vi "HW Configuration Dialog.vi"(8 "error in (no error)":errorcluster, 11 "Settings in":T2={"Support"={"Save Configuration"={"Log File Base Path"=path "", "TDMS File Reference"=refnum, "Reset"=FALSE, "Wait"=0.0, "Start Time"=0.0, "Update Rate"=1, "Channel Names"=[], "System Preset"=variant}, "LOG Configuration"={"LOG REF"=refnum, "Writer Queue"=refnum, "Log Path"=path "", "LOG"=FALSE}, "ALARM Configuration"={"LOG REF"=refnum, "Writer Queue"=refnum, "Log Path"=path "", "UPS standby"=FALSE, "status code"=5001, "SP"=[], "Over Sens Status"=[]}, "User Details"=[], "Radome Type"="", "Timer Configuration"={"Wait"=0.0, "Next Step"="", "Writer Queue"=refnum, "Reset"=FALSE, "VISA resource"="", "Status"=[], "Valve Time"=[], "Timer queue"=refnum, "Current valve"=0, "Enable"=FALSE}}, "Process"={"Test Configuration"={"current Step"=0, "Wait"=0.0, "Next Step"="", "Writer Queue"=refnum, "Reset"=FALSE, "SEQ Time"=0, "General Reset"=FALSE, "Cycles"=0, "Status"=[], "Ready"=[], "Backward"=FALSE, "Current SP"=[], "System Preset"={"Test Configuration"={"Cycles"=0, "Z Up"=0.0, "SP List"=[], "Operator"="", "Point Delay"=0, "Z Up 2"=0.0, "Cleaning In"=0.0, "Cleaning Out"=0.0, "Cleaning Cycles"=0}, "Test_Start_date"=""}, "Test Type"=enum."Calibration", "Sample Count"=0, "Local Queues"={"Cycles queue"=refnum, "Step queue"=refnum, "RES Queue"=refnum, "Clean queue"=refnum, "PS Scan queue"=refnum}, "current Clean"=0, "PS Measure Plan"=[]}}, "Report Configuration"={"Test Setting"={"Test_Num"=0, "Test_ID"=0, "Proc_ID"=0, "Max Force"=0.0, "User"="", "SN"="", "Date"=""}, "Measurements"=[], "LOG REF"=refnum, "Report Template"=path "", "Save Report path"=path "", "Data File Path"=path "", "Popup Dialog"=FALSE}, "History Data"={"Tests"=[], "Test Name"=""}, "Motor Configuration"={"Tango HW"={"VISA resource"="", "Baud Rate (115200)"=2, "lAnInterfaceType"=0, "bAShowProt"=15}, "Writer Queue"=refnum, "Status"=FALSE, "Abs Position"=[], "Axis Velocity"={"dX"=0.0, "dY"=0.0, "dZ"=0.0, "dA"=0.0}, "acceleration "=0.0, "Z direction"=enum."Up", "Position Mode"="", "plLSID"=0}, "PalmSense  Configuration"={"PalmSens.lvclass"=refnum, "Writer Queue"=refnum, "Enable"=FALSE, "Is Measuring Ref"=refnum, "Method"={"Name"="", "Method Ref"=variant}, "PS Live Curve Result"=refnum}, "Hiden Scanner Resources"={"Link"={"Connection"=enum."USB", "Host or IP address (TCP/IP)"="", "Port (Serial/USB)"="COM1"}, "VISA resource"="", "Writer Queue"=refnum, "Status"=FALSE}, "MFC Configuration"={"MFC Definition"={"MFC Port"="", "MFC Enable"=TRUE, "Baud Rate"=0, "Interface type"=enum."RS-485", "Address"=0}, "Set Point Options"={"Setpoint Value"=0.0, "Mass Flow EU 2"="", "Setpoint Source"="", "Valve Mode"=""}, "Writer Queue"=refnum, "Enable"=FALSE, "Update Rate"=0, "MRC Chamber Enable"=FALSE, "Selected Gas"="", "Address String"=""}, "Pump Configuration"={"Pump  name"=[], "Writer Queue"=refnum, "Pump Info"={"Pump Type"="", "Speed"=0, "Direction"=0, "Running"=FALSE}, "Current Pump Name"="", "Wait"=0.0, "Next Step"="", "Reset"=FALSE}} {"Pump Configuration"."Pump Info"."Direction" items=["CW", "CCW"]; "Pump Configuration"."Pump Info"."Speed" format="%03.0f"; "MFC Configuration"."Set Point Options"."Setpoint Value" min=0.0 max=0.62495 format="%.5f"; "Process"."Test Configuration"."PS Measure Plan" items=["Pretreatment settings (PS)", "Linear Sweep Voltammetry (LSV)", "Differential Pulse Voltammetry (DPV)", "Cyclic Voltammetry (CV)", "Chronoamperometry (CA)", "Chronopotentiometry (CP)", "El Imp Spectroscopy (EIS)"]; "Process"."Test Configuration"."System Preset"."Test Configuration"."SP List" format="%#.1g"; "Support"."Save Configuration"."Update Rate" min=1 max=10 step=1}) -> (0 "error out":errorcluster, 1 "Cancelled?":bool, 2 "UI Refresh Needed?":bool, 3 "Settings out":T2={"Support"={"Save Configuration"={"Log File Base Path"=path "", "TDMS File Reference"=refnum, "Reset"=FALSE, "Wait"=0.0, "Start Time"=0.0, "Update Rate"=1, "Channel Names"=[], "System Preset"=variant}, "LOG Configuration"={"LOG REF"=refnum, "Writer Queue"=refnum, "Log Path"=path "", "LOG"=FALSE}, "ALARM Configuration"={"LOG REF"=refnum, "Writer Queue"=refnum, "Log Path"=path "", "UPS standby"=FALSE, "status code"=5001, "SP"=[], "Over Sens Status"=[]}, "User Details"=[], "Radome Type"="", "Timer Configuration"={"Wait"=0.0, "Next Step"="", "Writer Queue"=refnum, "Reset"=FALSE, "VISA resource"="", "Status"=[], "Valve Time"=[], "Timer queue"=refnum, "Current valve"=0, "Enable"=FALSE}}, "Process"={"Test Configuration"={"current Step"=0, "Wait"=0.0, "Next Step"="", "Writer Queue"=refnum, "Reset"=FALSE, "SEQ Time"=0, "General Reset"=FALSE, "Cycles"=0, "Status"=[], "Ready"=[], "Backward"=FALSE, "Current SP"=[], "System Preset"={"Test Configuration"={"Cycles"=0, "Z Up"=0.0, "SP List"=[], "Operator"="", "Point Delay"=0, "Z Up 2"=0.0, "Cleaning In"=0.0, "Cleaning Out"=0.0, "Cleaning Cycles"=0}, "Test_Start_date"=""}, "Test Type"=enum."Calibration", "Sample Count"=0, "Local Queues"={"Cycles queue"=refnum, "Step queue"=refnum, "RES Queue"=refnum, "Clean queue"=refnum, "PS Scan queue"=refnum}, "current Clean"=0, "PS Measure Plan"=[]}}, "Report Configuration"={"Test Setting"={"Test_Num"=0, "Test_ID"=0, "Proc_ID"=0, "Max Force"=0.0, "User"="", "SN"="", "Date"=""}, "Measurements"=[], "LOG REF"=refnum, "Report Template"=path "", "Save Report path"=path "", "Data File Path"=path "", "Popup Dialog"=FALSE}, "History Data"={"Tests"=[], "Test Name"=""}, "Motor Configuration"={"Tango HW"={"VISA resource"="", "Baud Rate (115200)"=2, "lAnInterfaceType"=0, "bAShowProt"=15}, "Writer Queue"=refnum, "Status"=FALSE, "Abs Position"=[], "Axis Velocity"={"dX"=0.0, "dY"=0.0, "dZ"=0.0, "dA"=0.0}, "acceleration "=0.0, "Z direction"=enum."Up", "Position Mode"="", "plLSID"=0}, "PalmSense  Configuration"={"PalmSens.lvclass"=refnum, "Writer Queue"=refnum, "Enable"=FALSE, "Is Measuring Ref"=refnum, "Method"={"Name"="", "Method Ref"=variant}, "PS Live Curve Result"=refnum}, "Hiden Scanner Resources"={"Link"={"Connection"=enum."USB", "Host or IP address (TCP/IP)"="", "Port (Serial/USB)"="COM1"}, "VISA resource"="", "Writer Queue"=refnum, "Status"=FALSE}, "MFC Configuration"={"MFC Definition"={"MFC Port"="", "MFC Enable"=TRUE, "Baud Rate"=0, "Interface type"=enum."RS-485", "Address"=0}, "Set Point Options"={"Setpoint Value"=0.0, "Mass Flow EU 2"="", "Setpoint Source"="", "Valve Mode"=""}, "Writer Queue"=refnum, "Enable"=FALSE, "Update Rate"=0, "MRC Chamber Enable"=FALSE, "Selected Gas"="", "Address String"=""}, "Pump Configuration"={"Pump  name"=[], "Writer Queue"=refnum, "Pump Info"={"Pump Type"="", "Speed"=0, "Direction"=0, "Running"=FALSE}, "Current Pump Name"="", "Wait"=0.0, "Next Step"="", "Reset"=FALSE}} {"Pump Configuration"."Pump Info"."Direction" items=["CW", "CCW"]; "Pump Configuration"."Pump Info"."Speed" format="%03.0f"; "MFC Configuration"."Set Point Options"."Setpoint Value" min=0.0 max=0.62495 format="%.5f"; "Process"."Test Configuration"."PS Measure Plan" items=["Pretreatment settings (PS)", "Linear Sweep Voltammetry (LSV)", "Differential Pulse Voltammetry (DPV)", "Cyclic Voltammetry (CV)", "Chronoamperometry (CA)", "Chronopotentiometry (CP)", "El Imp Spectroscopy (EIS)"]; "Process"."Test Configuration"."System Preset"."Test Configuration"."SP List" format="%#.1g"; "Support"."Save Configuration"."Update Rate" min=1 max=10 step=1})   [LabVIEW 2020, in "Settings.lvlib"]
doc: "Dialog for selecting user specified settings."
uses:
  Settings.lvlib
  Settings.ctl
  <instrlib>/PalmSens SDK for LabVIEW 5.10/PalmSens/PalmSens.lvclass
  Logging/Save Configuration.ctl
  LOG/LOG Configuration.ctl
  support/Message Queue/Message Cluster.ctl
  ALARM/ALARM Configuration.ctl
  Valve Control/AM Configuration.ctl
  Test Driver/Test Driver Configuration.ctl
  Test Driver/System Preset.ctl
  Test Driver/Test Type.ctl
  Report/REP Configuration.ctl
  Report/Test Setting.ctl
  MOTOR/PS Hardware Configuration.ctl
  DMM/PalmSense Hardware Configuration.ctl
  Hiden Scanner/Scanner Hardware Configuration.ctl
  MRC/MRC Configuration.ctl
  WM Pump/Pump Hardware Configuration.ctl
  <vilib>/Utility/xml.llb/Write to XML File(string).vi
  Logging/SAVE.lvlib
  support/Message Queue/Message Queue.lvlib
  LOG/LOG.lvlib
  ALARM/QCT ALARM.lvlib
  Report/Report.lvlib
  MOTOR/MOTOR.lvlib
  Test Driver/Test Driver.lvlib
  DMM/PalmSens.lvlib
  Hiden Scanner/Hiden Scanner.lvlib
  Valve Control/Valve Control.lvlib
  MRC/MRC Module.lvlib
  WM Pump/Pump.lvlib
panel:
  in  "Instrument Definition":T1={"SYS XYZ Definition"={"Tango Port"="", "SYS 7000 Enable"=TRUE, "Baud Rate (57600)"=0, "Interface type"=0, "Show port"=0}, "Hiden Scanner Definition"={"Hiden Scanner VISA Name"="", "Hiden Enable"=TRUE, "Connection"=enum."USB"}, "Pump Definition"={"Pump VISA Name"="", "Pump Enable"=TRUE}, "MFC Definition"={"MFC Port"="", "MFC Enable"=TRUE, "Baud Rate"=0, "Interface type"=enum."RS-485", "Address"=0}, "PUMP name"=[], "Pump SET"={"Pump Type"="", "Speed"=0, "Direction"=0, "Running"=FALSE}} {"Pump SET"."Direction" items=["CW", "CCW"]; "Pump SET"."Speed" format="%03.0f"}
  out "power":bool
  in  "Cancel Button":bool
  in  "OK Button":bool
  # "Non visible portion of dialog (needed for connector pane)."
  # "Pump"
  # "In"
  # "Out"
  # "X"
  # "Y"
  # "Cycles"
  # "Point Delay"
  # "Up"
  # "Down"
  # "Z Axes"
  # "#C"
  # "In"
  # "Out"
  # "Cleaning [sec]"
  # "X"
  # "Y"
  # "Cycles"
  # "Point Delay"
  # "Up"
  # "Down"
  # "Z Axes"
  # "#C"
  # "In"
  # "Out"
  # "Cleaning [sec]"
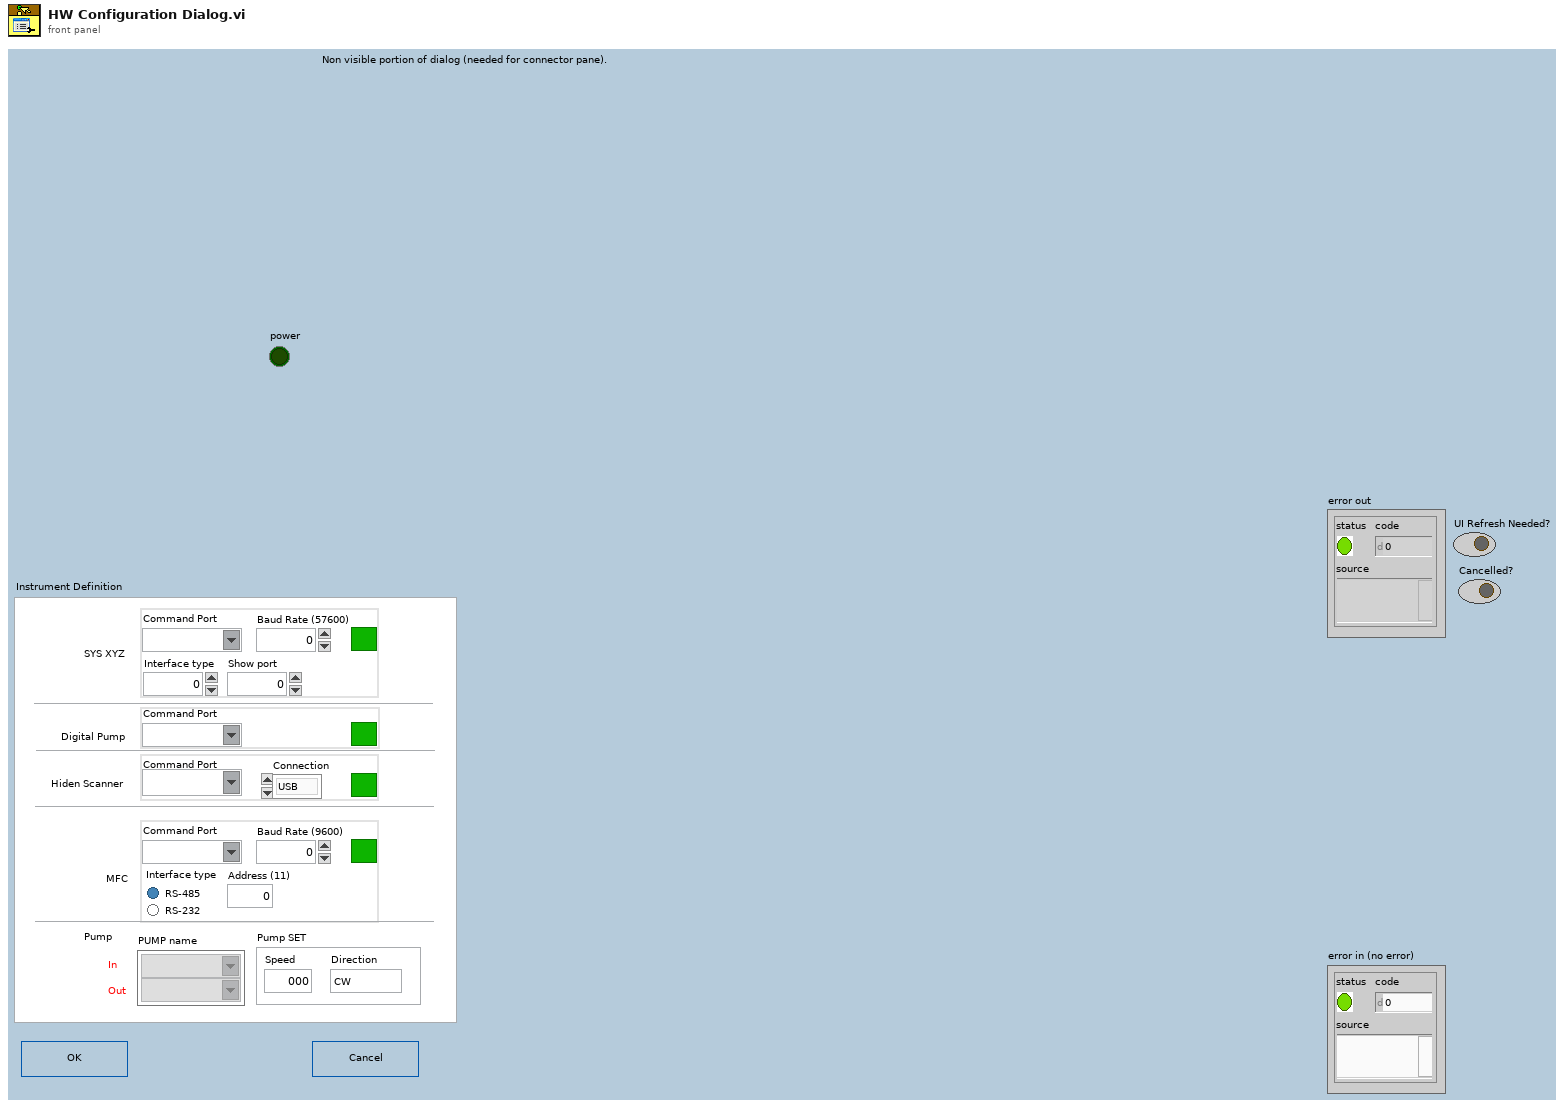
[diagram p1: front panel]
types:
  T1 = cluster{"SYS XYZ Definition":cluster{"Tango Port":refnum<visa-resource-name>, "SYS 7000 Enable":bool, "Baud Rate (57600)":i32, "Interface type":i32, "Show port":i32}, "Hiden Scanner Definition":cluster{"Hiden Scanner VISA Name":refnum<visa-resource-name>, "Hiden Enable":bool, "Connection":enum16{"Serial", "TCP/IP", "USB"}}, "Pump Definition":cluster{"Pump VISA Name":refnum<visa-resource-name>, "Pump Enable":bool}, "MFC Definition":cluster{"MFC Port":refnum<visa-resource-name>, "MFC Enable":bool, "Baud Rate":i32, "Interface type":enum32{"RS-485", "RS-232"}, "Address":i32}, "PUMP name":refnum<visa-resource-name>[], "Pump SET":cluster{"Pump Type":string, "Speed":i32, "Direction":u16, "Running":bool}}
  T2 = typedef "Settings.lvlib/Settings.ctl" = cluster{"Support":cluster{"Save Configuration":T3, "LOG Configuration":T4, "ALARM Configuration":T5, "User Details":string[], "Radome Type":string, "Timer Configuration":T6}, "Process":cluster{"Test Configuration":T7}, "Report Configuration":T10, "History Data":cluster{"Tests":string[][], "Test Name":string}, "Motor Configuration":T12, "PalmSense  Configuration":T13, "Hiden Scanner Resources":T14, "MFC Configuration":T15, "Pump Configuration":T16}
  T3 = typedef "SAVE.lvlib/Save Configuration.ctl" = cluster{"Log File Base Path":path, "TDMS File Reference":refnum<k34>, "Reset":bool, "Wait":dbl, "Start Time":dbl, "Update Rate":u16, "Channel Names":string[], "System Preset":variant}
  T4 = typedef "LOG.lvlib/LOG Configuration.ctl" = cluster{"LOG REF":refnum<vi>, "Writer Queue":refnum<queue>, "Log Path":path, "LOG":bool}
  T5 = typedef "QCT ALARM.lvlib/ALARM Configuration.ctl" = cluster{"LOG REF":refnum<vi>, "Writer Queue":refnum<queue>, "Log Path":path, "UPS standby":bool, "status code":i32, "SP":dbl[], "Over Sens Status":dbl[]}
  T6 = typedef "Valve Control.lvlib/AM Configuration.ctl" = cluster{"Wait":dbl, "Next Step":string, "Writer Queue":refnum<queue>, "Reset":bool, "VISA resource":refnum<visa-resource-name>, "Status":bool[], "Valve Time":dbl[], "Timer queue":refnum<queue>, "Current valve":i32, "Enable":bool}
  T7 = typedef "Test Driver.lvlib/Test Driver Configuration.ctl" = cluster{"current Step":i32, "Wait":dbl, "Next Step":string, "Writer Queue":refnum<queue>, "Reset":bool, "SEQ Time":i32, "General Reset":bool, "Cycles":i32, "Status":bool[], "Ready":bool[], "Backward":bool, "Current SP":dbl[], "System Preset":T8, "Test Type":T9, "Sample Count":i32, "Local Queues":cluster{"Cycles queue":refnum<queue>, "Step queue":refnum<queue>, "RES Queue":refnum<queue>, "Clean queue":refnum<queue>, "PS Scan queue":refnum<queue>}, "current Clean":i32, "PS Measure Plan":u16[]}
  T8 = typedef "System Preset.ctl" = cluster{"Test Configuration":cluster{"Cycles":i32, "Z Up":dbl, "SP List":dbl[][], "Operator":string, "Point Delay":i32, "Z Up 2":dbl, "Cleaning In":dbl, "Cleaning Out":dbl, "Cleaning Cycles":i32}, "Test_Start_date":string}
  T9 = typedef "Test Driver.lvlib/Test Type.ctl" = enum16{"Calibration", "Test"}
  T10 = typedef "Report.lvlib/REP Configuration.ctl" = cluster{"Test Setting":T11, "Measurements":string[][], "LOG REF":refnum<vi>, "Report Template":path, "Save Report path":path, "Data File Path":path, "Popup Dialog":bool}
  T11 = typedef "Report.lvlib/Test Setting.ctl" = cluster{"Test_Num":i32, "Test_ID":i32, "Proc_ID":i32, "Max Force":dbl, "User":string, "SN":string, "Date":string}
  T12 = typedef "MOTOR.lvlib/PS Hardware Configuration.ctl" = cluster{"Tango HW":cluster{"VISA resource":refnum<visa-resource-name>, "Baud Rate (115200)":i32, "lAnInterfaceType":i32, "bAShowProt":i32}, "Writer Queue":refnum<queue>, "Status":bool, "Abs Position":i32[], "Axis Velocity":cluster{"dX":dbl, "dY":dbl, "dZ":dbl, "dA":dbl}, "acceleration ":dbl, "Z direction":enum16{"Up", "Down"}, "Position Mode":string, "plLSID":i32}
  T13 = typedef "PalmSens.lvlib/PalmSense Hardware Configuration.ctl" = cluster{"PalmSens.lvclass":refnum<class "PalmSens.lvclass">, "Writer Queue":refnum<queue>, "Enable":bool, "Is Measuring Ref":refnum<vi>, "Method":cluster{"Name":string, "Method Ref":variant}, "PS Live Curve Result":refnum<vi>}
  T14 = typedef "Hiden Scanner.lvlib/Scanner Hardware Configuration.ctl" = cluster{"Link":cluster{"Connection":enum16{"Serial", "TCP/IP", "USB"}, "Host or IP address (TCP/IP)":string, "Port (Serial/USB)":string}, "VISA resource":refnum<visa-resource-name>, "Writer Queue":refnum<queue>, "Status":bool}
  T15 = typedef "MRC Module.lvlib/MRC Configuration.ctl" = cluster{"MFC Definition":cluster{"MFC Port":refnum<visa-resource-name>, "MFC Enable":bool, "Baud Rate":i32, "Interface type":enum32{"RS-485", "RS-232"}, "Address":i32}, "Set Point Options":cluster{"Setpoint Value":dbl, "Mass Flow EU 2":string, "Setpoint Source":string, "Valve Mode":string}, "Writer Queue":refnum<queue>, "Enable":bool, "Update Rate":u32, "MRC Chamber Enable":bool, "Selected Gas":string, "Address String":string}
  T16 = typedef "Pump.lvlib/Pump Hardware Configuration.ctl" = cluster{"Pump  name":refnum<visa-resource-name>[], "Writer Queue":refnum<queue>, "Pump Info":cluster{"Pump Type":string, "Speed":i32, "Direction":u16, "Running":bool}, "Current Pump Name":refnum<visa-resource-name>, "Wait":dbl, "Next Step":string, "Reset":bool}
  T17 = cluster{"MFC Port":refnum<visa-resource-name>, "MFC Enable":bool, "Baud Rate":i32, "Interface type":enum32{"RS-485", "RS-232"}, "Address":i32}
  T18 = cluster{"Pump Type":string, "Speed":i32, "Direction":u16, "Running":bool}
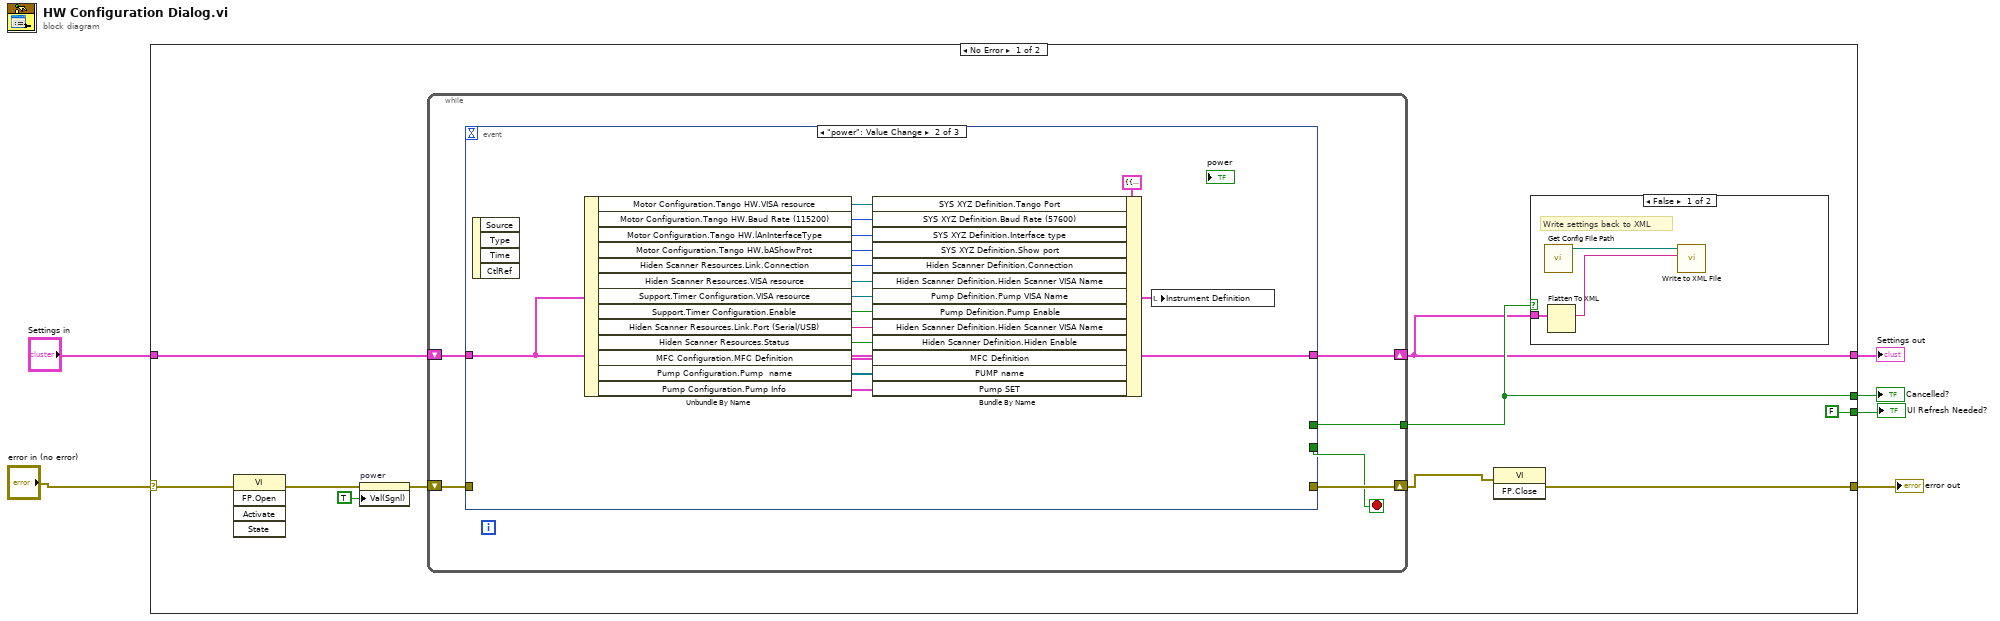
[diagram p0: block diagram]
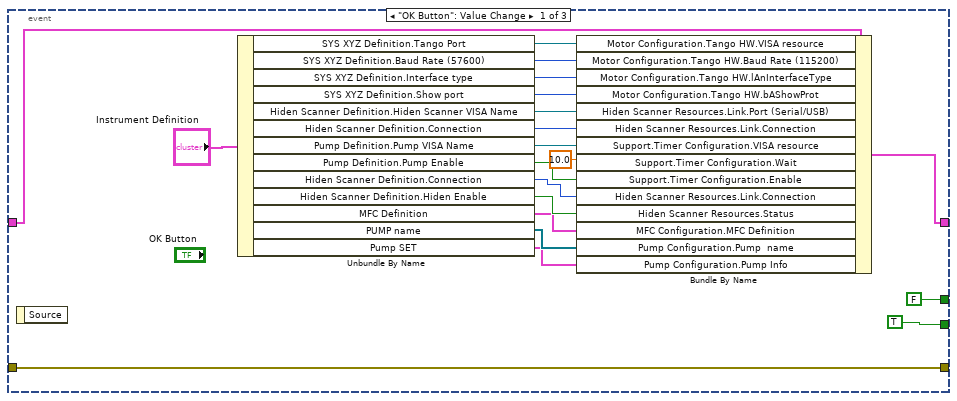
[diagram p2: hidden frame]
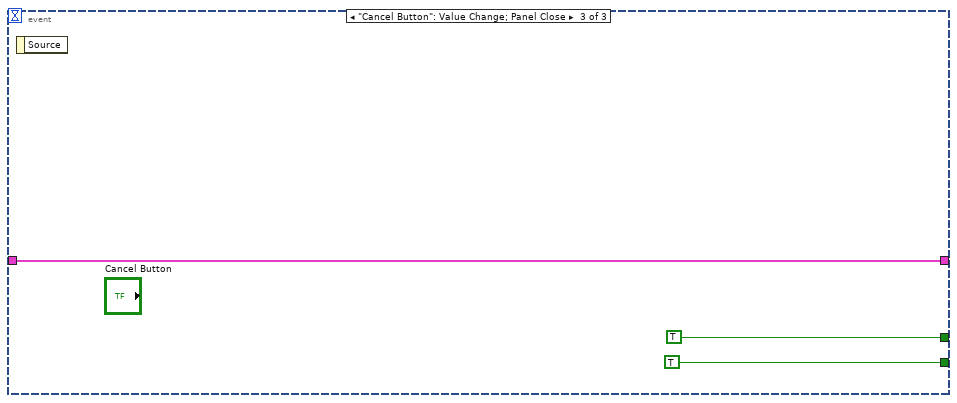
[diagram p3: hidden frame]
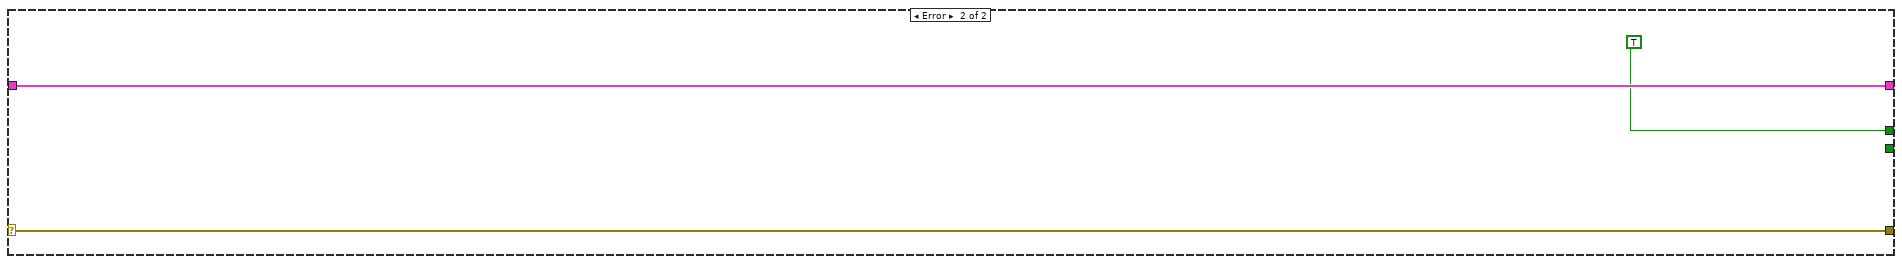
[diagram p5: hidden frame]
diagram:
  n1 = case shown="No Error" "error in (no error)" {
    selector: "error in (no error)" -> [w11 w67]
    tunnel: [w10 w67] -> w5
    tunnel: "Settings in" -> [w13 w66]
    tunnel: [w14 w66] -> w4
    tunnel: [FALSE ("UI Refresh Needed?") _] -> w3
    tunnel: [w15 TRUE ("UI Refresh Needed?")] -> w2
    frame No Error {
      n2 = invoke class="VI" method="FP.Open"(error in=w11) -> (error out=w9:errorcluster)  [unwired: 4 in, 4 out]
      n3 = property on="power" class="Bool (strict)"(error in=w9, "Val(Sgnl)"=TRUE ("Value (Signaling)")) -> (error out=w7:errorcluster)  [unwired: 1 in, 1 out]
      n4 = while {
        tunnel: [w18] -> w15
        shift-right: [w22] -> w14
        shift-left: w13 -> [w21]
        shift-right: [w19] -> w12
        shift-left: w7 -> [w20]
        stop <- w17 stop-if-true
        n5 = event shown="[1] \"power\": Value Change" {
          selector: _ -> [_ _ _]
          dyn-events: _ -> [_ _ _]
          timeout: _ -> [_ _ _]
          tunnel: [w38 w58 w61] -> w22
          tunnel: w21 -> [w41 w58 w61]
          tunnel: [FALSE ("UI Refresh Needed?") _ TRUE ("UI Refresh Needed?")] -> w18
          tunnel: w20 -> [w40 _ _]
          tunnel: [w40 _ _] -> w19
          tunnel: [TRUE _ TRUE] -> w17
          event "OK Button": Value Change {
            n6 = event-data() -> ()  [unwired: 1 in, 1 out]
            n7 = Unbundle By Name("Instrument Definition") -> ("SYS XYZ Definition.Tango Port"=w36:refnum<visa-resource-name>, "SYS XYZ Definition.Baud Rate (57600)"=w35:i32, "SYS XYZ Definition.Interface type"=w33:i32, "SYS XYZ Definition.Show port"=w32:i32, "Hiden Scanner Definition.Hiden Scanner VISA Name"=w34:refnum<visa-resource-name>, "Hiden Scanner Definition.Connection"=w31:enum16{"Serial", "TCP/IP", "USB"}, "Pump Definition.Pump VISA Name"=w30:refnum<visa-resource-name>, "Pump Definition.Pump Enable"=w28:bool, "Hiden Scanner Definition.Connection"=w27:enum16{"Serial", "TCP/IP", "USB"}, "Hiden Scanner Definition.Hiden Enable"=w26:bool, "MFC Definition"=w25:T17, "PUMP name"=w24:refnum<visa-resource-name>[], "Pump SET"=w23:T18)
            n8 = Bundle By Name(cluster=w41, "Motor Configuration.Tango HW.VISA resource"=w36, "Motor Configuration.Tango HW.Baud Rate (115200)"=w35, "Motor Configuration.Tango HW.lAnInterfaceType"=w33, "Motor Configuration.Tango HW.bAShowProt"=w32, "Hiden Scanner Resources.Link.Port (Serial/USB)"=w34, "Hiden Scanner Resources.Link.Connection"=w31, "Support.Timer Configuration.VISA resource"=w30, "Support.Timer Configuration.Wait"=10.0, "Support.Timer Configuration.Enable"=w28, "Hiden Scanner Resources.Link.Connection"=w27, "Hiden Scanner Resources.Status"=w26, "MFC Configuration.MFC Definition"=w25, "Pump Configuration.Pump  name"=w24, "Pump Configuration.Pump Info"=w23) -> (w38:T2)
          }
          event "power": Value Change {
            n9 = event-data() -> ()  [unwired: 1 in, 4 out]
            n10 = Unbundle By Name(w58) -> ("Motor Configuration.Tango HW.VISA resource"=w57:refnum<visa-resource-name>, "Motor Configuration.Tango HW.Baud Rate (115200)"=w56:i32, "Motor Configuration.Tango HW.lAnInterfaceType"=w55:i32, "Motor Configuration.Tango HW.bAShowProt"=w54:i32, "Hiden Scanner Resources.Link.Connection"=w53:enum16{"Serial", "TCP/IP", "USB"}, "Hiden Scanner Resources.VISA resource"=w52:refnum<visa-resource-name>, "Support.Timer Configuration.VISA resource"=w50:refnum<visa-resource-name>, "Support.Timer Configuration.Enable"=w49:bool, "Hiden Scanner Resources.Link.Port (Serial/USB)"=w48:string, "Hiden Scanner Resources.Status"=w47:bool, "MFC Configuration.MFC Definition"=w46:T17, "Pump Configuration.Pump  name"=w45:refnum<visa-resource-name>[], "Pump Configuration.Pump Info"=w44:T18)
            n11 = Bundle By Name(cluster=T1 {"SYS XYZ Definition"={"Tango Port"="COM7", "SYS 7000 Enable"=TRUE, "Baud Rate (57600)"=57600, "Interface type"=1, "Show port"=1}, "Hiden Scanner Definition"={"Hiden Scanner VISA Name"="COM9", "Hiden Enable"=TRUE, "Connection"=enum."USB"}, "Pump Definition"={"Pump VISA Name"="COM14", "Pump Enable"=TRUE}, "MFC Definition"={"MFC Port"="COM16", "MFC Enable"=TRUE, "Baud Rate"=9600, "Interface type"=enum."RS-232", "Address"=11}, "PUMP name"=[], "Pump SET"={"Pump Type"="", "Speed"=100, "Direction"=1, "Running"=FALSE}} ("Instrument Definition"), "SYS XYZ Definition.Tango Port"=w57, "SYS XYZ Definition.Baud Rate (57600)"=w56, "SYS XYZ Definition.Interface type"=w55, "SYS XYZ Definition.Show port"=w54, "Hiden Scanner Definition.Connection"=w53, "Hiden Scanner Definition.Hiden Scanner VISA Name"=w52, "Pump Definition.Pump VISA Name"=w50, "Pump Definition.Pump Enable"=w49, "Hiden Scanner Definition.Hiden Scanner VISA Name"=w48, "Hiden Scanner Definition.Hiden Enable"=w47, "MFC Definition"=w46, "PUMP name"=w45, "Pump SET"=w44) -> (w51:T1)
            n12 = local write "Instrument Definition"(w51) -> ()
          }
          event "Cancel Button": Value Change; Panel Close {
            n13 = event-data() -> ()  [unwired: 1 in, 1 out]
          }
        }
      }
      n14 = invoke class="VI" method="FP.Close"(error in=w12) -> (error out=w10:errorcluster)  [unwired: 2 in, 2 out]
      n15 = case shown="False" w15 {
        tunnel: w14 -> [w63 _]
        frame False {
          # "Write settings back to XML"
          n16 = call "Get Config File Path.vi"() -> ("XML File Path"=w64:path)  [unwired: 10 in, 1 out]
          n17 = Flatten To XML(6:w63) -> (2:w62:string)
          n18 = call-poly <vilib>:"Write to XML File.vi"("XML Input"=w62, "XML File Path"=w64) -> ()  [unwired: 7 in, 3 out]
        }
        frame True {
        }
      }
    }
    frame Error {
    }
  }
  "UI Refresh Needed?" <- w3
  "error out" <- w5
  "Settings out" <- w4
  "Cancelled?" <- w2
